vi "Helper SubVI - Online Plot Detrend Signal.vi"(7 "initialize? (F)":bool, 9 "trend signal":dbl[](array[numeric]), 10 "detrended signal":dbl[](array[numeric]), 11 "signal":dbl[](array[numeric])) -> (1 "trend signal out":dbl[](array[numeric]), 2 "detrended signal out":dbl[](array[numeric]), 3 "signal out":dbl[](array[numeric]))   [LabVIEW 2023]
doc: "Generates online plots including the original signal, detrended signal, and trend signal."
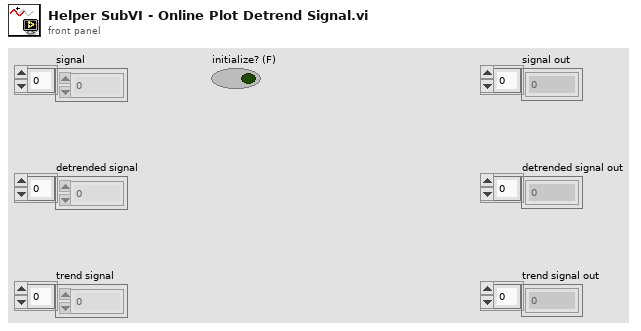
[diagram p1: front panel]
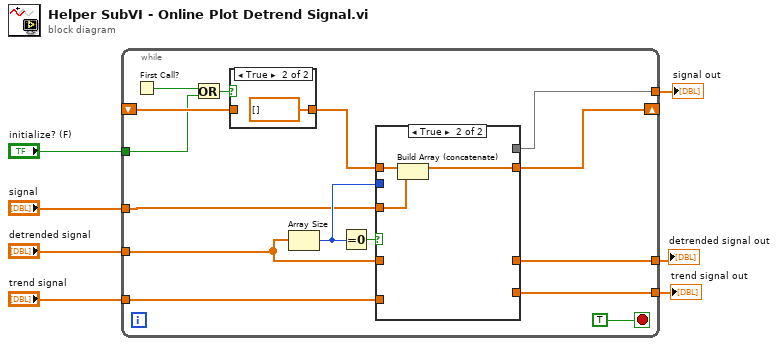
[diagram p0: block diagram]
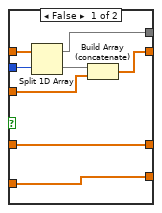
[diagram p3: hidden frame]
diagram:
  n1 = while {
    shift-right: [w22] -> _
    shift-left: _ -> [w18]
    tunnel: "initialize? (F)" -> [w14]
    tunnel: "signal" -> [w13]
    tunnel: "detrended signal" -> [w12]
    tunnel: "trend signal" -> [w11]
    tunnel: [w10] -> w3
    tunnel: [w9] -> w2
    tunnel: [w8] -> w1
    stop <- TRUE stop-if-true
    n2 = First Call?() -> (First Call?: T/F=w16:bool)
    n3 = Or(x=w16, y=w14) -> (x .or. y?=w15:bool)
    n4 = case shown="True" w15 {
      tunnel: w18 -> [w23 _]
      tunnel: [w23 dbl[] []] -> w17
      frame False {
      }
      frame True {
      }
    }
    n5 = Array Size(array=w12) -> (size(s)=w20:i32)
    n6 = Equal To 0?(x=w20) -> (x = 0?=w21:bool)
    n7 = case shown="True" w21 {
      tunnel: [w31 w33] -> w22
      tunnel: w17 -> [w28 w35]
      tunnel: w13 -> [w32 w34]
      tunnel: w20 -> [w27 _]
      tunnel: w12 -> [w30 _]
      tunnel: [w30 _] -> w9
      tunnel: w11 -> [w29 _]
      tunnel: [w29 _] -> w8
      tunnel: [w25 _] -> w10
      frame False {
        n8 = Split 1D Array(array=w28, index=w27) -> (first subarray=w25:dbl[], second subarray=w26:dbl[])
        n9 = Build Array (concatenate)(w26, w32) -> (w31:dbl[])
      }
      frame True {
        n10 = Build Array (concatenate)(w35, w34) -> (w33:dbl[])
      }
    }
  }
  "signal out" <- w3
  "detrended signal out" <- w2
  "trend signal out" <- w1
